vi "sv_Swept Sine Apply Window (dual).vi"(4 "read/write indices":T1(array[cluster]), 6 "AI index":i32, 7 "reset phase":bool, 11 "data to process":cluster{"stimulus":dbl[], "response":dbl[]} {"response" format="%.2f"; "stimulus" format="%.2f"}) -> (1 "ENBW":dbl=90.0 format="%.2f", 3 "windowed data":cluster{"stimulus":dbl[], "response":dbl[]} {"response" format="%.2f"; "stimulus" format="%.2f"})   [LabVIEW 2017, in "SoundVib_SweptSine.lvlib"]
uses:
  <vilib>/addons/Sound and Vibration/svt_Swept Sine/SoundVib_SweptSine.lvlib
  <vilib>/Analysis/NI_AALBase.lvlib
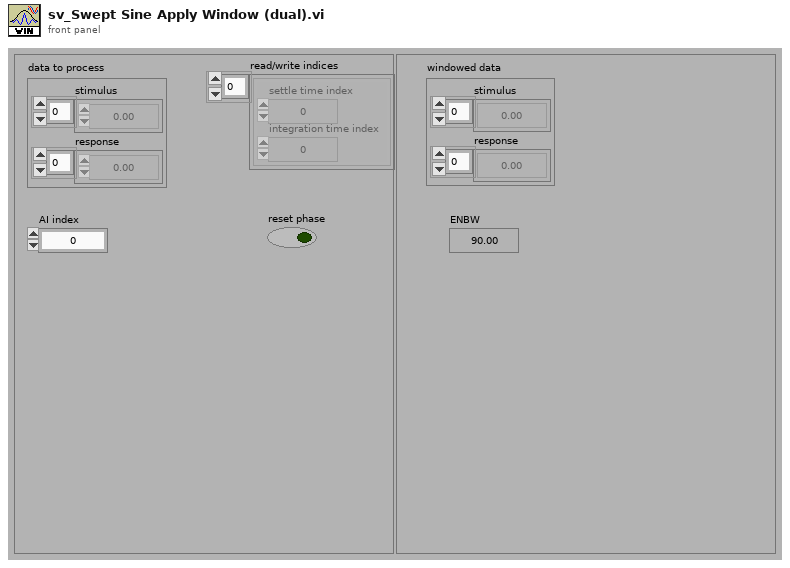
[diagram p1: front panel]
types:
  T1 = cluster{"settle time index":u32, "integration time index":u32}[]
  T2 = cluster{"settle time index":u32, "integration time index":u32}
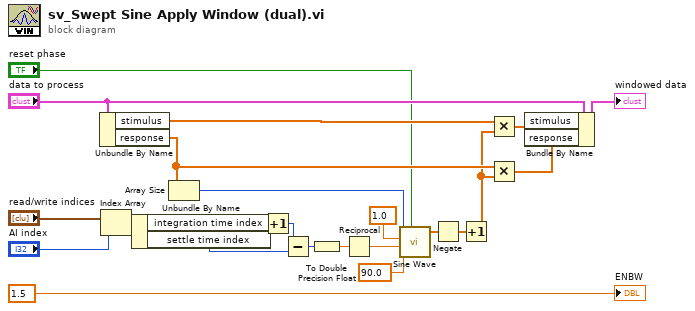
[diagram p0: block diagram]
diagram:
  n1 = Unbundle By Name("data to process") -> ("stimulus"=w19:dbl[], "response"=w18:dbl[])
  n2 = Index Array(array="read/write indices", index="AI index") -> (element=w9:T2)
  n3 = Unbundle By Name(w9) -> ("integration time index"=w12:u32, "settle time index"=w10:u32)
  n4 = Array Size(array=w18) -> (size(s)=w7:i32)
  n5 = Increment(x=w12) -> (x+1=w11:u32)
  n6 = Subtract(x=w11, y=w10) -> (x-y=w14:u32)
  n7 = To Double Precision Float(number=w14) -> (double precision float=w8:dbl)
  n8 = Reciprocal(x=w8) -> (1/x=w13:dbl)
  n9 = call <vilib>:"Sine Wave.vi"("samples"=w7, "amplitude"=1.0, "frequency"=w13, "phase in"=90.0, "reset phase"="reset phase") -> ("sine wave"=w17:dbl[])  [unwired: 2 out]
  n10 = Negate(x=w17) -> (-x=w16:dbl[])
  n11 = Increment(x=w16) -> (x+1=w6:dbl[])
  n12 = Multiply(x=w19, y=w6) -> (x*y=w20:dbl[])
  n13 = Multiply(x=w18, y=w6) -> (x*y=w21:dbl[])
  n14 = Bundle By Name(cluster="data to process", "stimulus"=w20, "response"=w21) -> (→"windowed data":cluster{"stimulus":dbl[], "response":dbl[]})
  "ENBW" <- 1.5 ("ENBW")
